vi "Open Plugin gRPC.vi"(6 "Server Certificate File (.crt)":path, 8 "error in (no error)":errorcluster, 9 "Type":string, 10 "address":string, 11 "CIF_UI in":refnum<class "CIF_UI.lvclass">) -> (0 "error out":errorcluster, 2 "gRPC ID Out":T1, 3 "CIF_UI out":refnum<class "CIF_UI.lvclass">)   [LabVIEW 2021, in "CIF_UI.lvclass"]
uses:
  CIF_UI.lvclass
  <vilib>/gRPC/LabVIEW gRPC Library/Shared/grpcId.ctl
  CIFCore/Grpc/CIFCoreWrapper/CIFCoreWrapper.lvlib
  <vilib>/gRPC/LabVIEW gRPC Library/grpc-lvsupport-release.lvlib
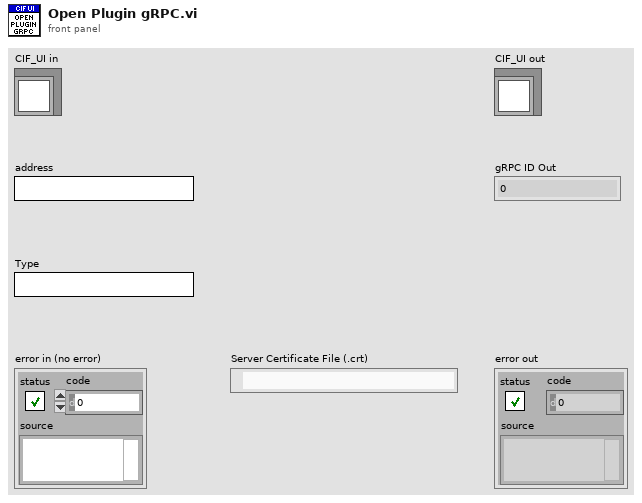
[diagram p1: front panel]
types:
  T1 = typedef "grpc-lvsupport-release.lvlib/grpcId.ctl" = u64
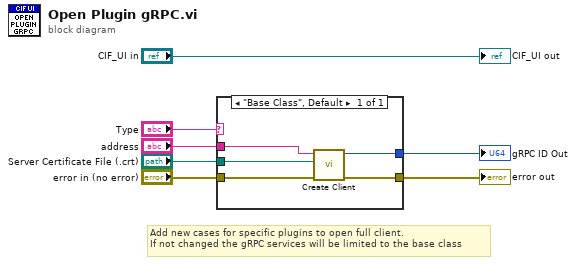
[diagram p0: block diagram]
diagram:
  # "Add new cases for specific plugins to open full client.\nIf not changed the gRPC services will be limited to the base class"
  n1 = case shown="\"Base Class\", Default" "Type" {
    tunnel: "error in (no error)" -> [w12]
    tunnel: [w11] -> w5
    tunnel: [w10] -> w4
    tunnel: "address" -> [w9]
    tunnel: "Server Certificate File (.crt)" -> [w8]
    frame "Base Class", Default {
      n2 = call "Create Client.vi"("error in"=w12, "Server Certificate File (.crt)"=w8, "address"=w9) -> ("error out"=w11:errorcluster, "gRPC ID Out"=w10:T1)  [unwired: 7 in]
    }
  }
  "error out" <- w5
  "gRPC ID Out" <- w4
  "CIF_UI out" <- "CIF_UI in"
